vi "GetProbePlanCoordinates.vi"(8 "Use index as X coord":bool=TRUE, 9 "Probe Card Channels":i32=1) -> (0 "file path":string, 2 "OK?":bool, 3 "Array":T1(array[cluster]))   [LabVIEW 2018] (continued)
y=33870.77 \nLabel=Strip\t1026\tX=71822.91\ty=33981.80 \nLabel=Strip\t1027\tX=71468.59\ty=34027.48 \nLabel=Strip\t1028\tX=71811.19\ty=34138.63 \nLabel=Strip\t1029\tX=71456.86\ty=34184.19 \nLabel=Strip\t1030\tX=71799.42\ty=34295.46 \nLabel=Strip\t1031\tX=71445.07\ty=34340.89 \nLabel=Strip\t1032\tX=71787.60\ty=34452.28 \nLabel=Strip\t1033\tX=71433.24\ty=34497.60 \nLabel=Strip\t1034\tX=71775.72\ty=34609.10 \nLabel=Strip\t1035\tX=71421.34\ty=34654.30 \nLabel=Strip\t1036\tX=71763.79\ty=34765.92 \nLabel=Strip\t1037\tX=71409.40\ty=34810.99 \nLabel=Strip\t1038\tX=71751.81\ty=34922.74 \nLabel=Strip\t1039\tX=71397.40\ty=34967.69 \nLabel=Strip\t1040\tX=71739.77\ty=35079.55 \nLabel=Strip\t1041\tX=71385.34\ty=35124.38 \nLabel=Strip\t1042\tX=71727.67\ty=35236.35 \nLabel=Strip\t1043\tX=71373.23\ty=35281.06 \nLabel=Strip\t1044\tX=71715.53\ty=35393.16 \nLabel=Strip\t1045\tX=71361.07\ty=35437.75 \nLabel=Strip\t1046\tX=71703.33\ty=35549.96 \nLabel=Strip\t1047\tX=71348.85\ty=35594.43 \nLabel=Strip\t1048\tX=71691.07\ty=35706.76 \nLabel=Strip\t1049\tX=71336.58\ty=35751.10 \nLabel=Strip\t1050\tX=71678.76\ty=35863.56 \nLabel=Strip\t1051\tX=71324.26\ty=35907.78 \nLabel=Strip\t1052\tX=71666.40\ty=36020.35 \nLabel=Strip\t1053\tX=71311.88\ty=36064.45 \nLabel=Strip\t1054\tX=71653.98\ty=36177.14 \nLabel=Strip\t1055\tX=71299.45\ty=36221.12 \nLabel=Strip\t1056\tX=71641.51\ty=36333.92 \nLabel=Strip\t1057\tX=71286.96\ty=36377.78 \nLabel=Strip\t1058\tX=71628.98\ty=36490.71 \nLabel=Strip\t1059\tX=71274.42\ty=36534.44 \nLabel=Strip\t1060\tX=71616.41\ty=36647.49 \nLabel=Strip\t1061\tX=71261.83\ty=36691.10 \nLabel=Strip\t1062\tX=71603.77\ty=36804.26 \nLabel=Strip\t1063\tX=71249.18\ty=36847.76 \nLabel=Strip\t1064\tX=71591.09\ty=36961.03 \nLabel=Strip\t1065\tX=71236.48\ty=37004.41 \nLabel=Strip\t1066\tX=71578.34\ty=37117.80 \nLabel=Strip\t1067\tX=71223.72\ty=37161.06 \nLabel=Strip\t1068\tX=71565.55\ty=37274.57 \nLabel=Strip\t1069\tX=71210.91\ty=37317.70 \nLabel=Strip\t1070\tX=71552.70\ty=37431.33 \nLabel=Strip\t1071\tX=71198.05\ty=37474.34 \nLabel=Strip\t1072\tX=71539.80\ty=37588.09 \nLabel=Strip\t1073\tX=71185.13\ty=37630.98 \nLabel=Strip\t1074\tX=71526.84\ty=37744.85 \nLabel=Strip\t1075\tX=71172.16\ty=37787.61 \nLabel=Strip\t1076\tX=71513.83\ty=37901.60 \nLabel=Strip\t1077\tX=71159.13\ty=37944.25 \nLabel=Strip\t1078\tX=71500.76\ty=38058.35 \nLabel=Strip\t1079\tX=71146.05\ty=38100.87 \nLabel=Strip\t1080\tX=71487.64\ty=38215.09 \nLabel=Strip\t1081\tX=71132.92\ty=38257.50 \nLabel=Strip\t1082\tX=71474.47\ty=38371.83 \nLabel=Strip\t1083\tX=71119.73\ty=38414.12 \nLabel=Strip\t1084\tX=71461.24\ty=38528.57 \nLabel=Strip\t1085\tX=71106.49\ty=38570.73 \nLabel=Strip\t1086\tX=71447.96\ty=38685.31 \nLabel=Strip\t1087\tX=71093.19\ty=38727.35 \nLabel=Strip\t1088\tX=71434.62\ty=38842.04 \nLabel=Strip\t1089\tX=71079.84\ty=38883.96 \nLabel=Strip\t1090\tX=71421.24\ty=38998.77 \nLabel=Strip\t1091\tX=71066.44\ty=39040.56 \nLabel=Strip\t1092\tX=71407.79\ty=39155.49 \nLabel=Strip\t1093\tX=71052.98\ty=39197.17 \nLabel=Strip\t1094\tX=71394.30\ty=39312.21 \nLabel=Strip\t1095\tX=71039.47\ty=39353.77 \nLabel=Strip\t1096\tX=71380.74\ty=39468.93 \nLabel=Strip\t1097\tX=71025.90\ty=39510.36 \nLabel=Strip\t1098\tX=71367.14\ty=39625.64 \nLabel=Strip\t1099\tX=71012.28\ty=39666.95 \nLabel=Strip\t1100\tX=71353.48\ty=39782.35 \nLabel=Strip\t1101\tX=70998.61\ty=39823.54 \nLabel=Strip\t1102\tX=71339.77\ty=39939.06 \nLabel=Strip\t1103\tX=70984.88\ty=39980.13 \nLabel=Strip\t1104\tX=71326.00\ty=40095.76 \nLabel=Strip\t1105\tX=70971.10\ty=40136.71 \nLabel=Strip\t1106\tX=71312.18\ty=40252.46 \nLabel=Strip\t1107\tX=70957.26\ty=40293.29 \nLabel=Strip\t1108\tX=71298.30\ty=40409.15 \nLabel=Strip\t1109\tX=70943.37\ty=40449.86 \nLabel=Strip\t1110\tX=71284.37\ty=40565.84 \nLabel=Strip\t1111\tX=70929.43\ty=40606.43 \nLabel=Strip\t1112\tX=71270.39\ty=40722.53 \nLabel=Strip\t1113\tX=70915.43\ty=40762.99 \nLabel=Strip\t1114\tX=71256.35\ty=40879.21 \nLabel=Strip\t1115\tX=70901.38\ty=40919.56 \nLabel=Strip\t1116\tX=71242.26\ty=41035.89 \nLabel=Strip\t1117\tX=70887.28\ty=41076.11 \nLabel=Strip\t1118\tX=71228.11\ty=41192.57 \nLabel=Strip\t1119\tX=70873.12\ty=41232.67 \nLabel=Strip\t1120\tX=71213.92\ty=41349.24 \nLabel=Strip\t1121\tX=70858.90\ty=41389.22 \nLabel=Strip\t1122\tX=71199.66\ty=41505.91 \nLabel=Strip\t1123\tX=70844.64\ty=41545.77 \nLabel=Strip\t1124\tX=71185.36\ty=41662.57 \nLabel=Strip\t1125\tX=70830.32\ty=41702.31 \nLabel=Strip\t1126\tX=71170.99\ty=41819.23 \nLabel=Strip\t1127\tX=70815.94\ty=41858.85 \nLabel=Strip\t1128\tX=71156.58\ty=41975.89 \nLabel=Strip\t1129\tX=70801.51\ty=42015.38 \nLabel=Strip\t1130\tX=71142.11\ty=42132.54 \nLabel=Strip\t1131\tX=70787.03\ty=42171.91 \nLabel=Strip\t1132\tX=71127.59\ty=42289.19 \nLabel=Strip\t1133\tX=70772.49\ty=42328.44 \nLabel=Strip\t1134\tX=71113.01\ty=42445.83 \nLabel=Strip\t1135\tX=70757.90\ty=42484.96 \nLabel=Strip\t1136\tX=71098.38\ty=42602.47 \nLabel=Strip\t1137\tX=70743.26\ty=42641.48 \nLabel=Strip\t1138\tX=71083.69\ty=42759.11 \nLabel=Strip\t1139\tX=70728.56\ty=42798.00 \nLabel=Strip\t1140\tX=71068.95\ty=42915.74 \nLabel=Strip\t1141\tX=70713.80\ty=42954.51 \nLabel=Strip\t1142\tX=71054.16\ty=43072.37 \nLabel=Strip\t1143\tX=70699.00\ty=43111.01 \nLabel=Strip\t1144\tX=71039.31\ty=43229.00 \nLabel=Strip\t1145\tX=70684.14\ty=43267.52 \nLabel=Strip\t1146\tX=71024.41\ty=43385.62 \nLabel=Strip\t1147\tX=70669.22\ty=43424.02 \nLabel=Strip\t1148\tX=71009.46\ty=43542.23 \nLabel=Strip\t1149\tX=70654.25\ty=43580.51 \nLabel=Strip\t1150\tX=70994.45\ty=43698.84 \nLabel=Strip\t1151\tX=70639.23\ty=43737.00 \nLabel=Strip\t1152\tX=70979.38\ty=43855.45 \nLabel=Strip\t1153\tX=70624.16\ty=43893.49 \nLabel=Strip\t1154\tX=70964.27\ty=44012.06 \nRegion=Segment\t0T\nLabel=Strip\t1\tX=100771.56\ty=-48853.60 \nLabel=Strip\t2\tX=101128.74\ty=-48799.25 \nLabel=Strip\t3\tX=100788.28\ty=-48687.35 \nLabel=Strip\t4\tX=101145.44\ty=-48632.88 \nLabel=Strip\t5\tX=100804.94\ty=-48521.10 \nLabel=Strip\t6\tX=101162.09\ty=-48466.50 \nLabel=Strip\t7\tX=100821.55\ty=-48354.83 \nLabel=Strip\t8\tX=101178.67\ty=-48300.12 \nLabel=Strip\t9\tX=100838.10\ty=-48188.57 \nLabel=Strip\t10\tX=101195.20\ty=-48133.73 \nLabel=Strip\t11\tX=100854.59\ty=-48022.29 \nLabel=Strip\t12\tX=101211.68\ty=-47967.33 \nLabel=Strip\t13\tX=100871.02\ty=-47856.01 \nLabel=Strip\t14\tX=101228.10\ty=-47800.92 \nLabel=Strip\t15\tX=100887.40\ty=-47689.72 \nLabel=Strip\t16\tX=101244.45\ty=-47634.51 \nLabel=Strip\t17\tX=100903.72\ty=-47523.43 \nLabel=Strip\t18\tX=101260.76\ty=-47468.10 \nLabel=Strip\t19\tX=100919.99\ty=-47357.13 \nLabel=Strip\t20\tX=101277.00\ty=-47301.67 \nLabel=Strip\t21\tX=100936.20\ty=-47190.82 \nLabel=Strip\t22\tX=101293.19\ty=-47135.24 \nLabel=Strip\t23\tX=100952.35\ty=-47024.51 \nLabel=Strip\t24\tX=101309.32\ty=-46968.80 \nLabel=Strip\t25\tX=100968.44\ty=-46858.19 \nLabel=Strip\t26\tX=101325.40\ty=-46802.36 \nLabel=Strip\t27\tX=100984.48\ty=-46691.86 \nLabel=Strip\t28\tX=101341.41\ty=-46635.91 \nLabel=Strip\t29\tX=101000.46\ty=-46525.53 \nLabel=Strip\t30\tX=101357.37\ty=-46469.45 \nLabel=Strip\t31\tX=101016.38\ty=-46359.18 \nLabel=Strip\t32\tX=101373.28\ty=-46302.99 \nLabel=Strip\t33\tX=101032.25\ty=-46192.84 \nLabel=Strip\t34\tX=101389.13\ty=-46136.52 \nLabel=Strip\t35\tX=101048.05\ty=-46026.49 \nLabel=Strip\t36\tX=101404.91\ty=-45970.04 \nLabel=Strip\t37\tX=101063.81\ty=-45860.13 \nLabel=Strip\t38\tX=101420.65\ty=-45803.57 \nLabel=Strip\t39\tX=101079.50\ty=-45693.76 \nLabel=Strip\t40\tX=101436.32\ty=-45637.07 \nLabel=Strip\t41\tX=101095.14\ty=-45527.39 \nLabel=Strip\t42\tX=101451.94\ty=-45470.58 \nLabel=Strip\t43\tX=101110.72\ty=-45361.01 \nLabel=Strip\t44\tX=101467.50\ty=-45304.08 \nLabel=Strip\t45\tX=101126.24\ty=-45194.62 \nLabel=Strip\t46\tX=101483.01\ty=-45137.57 \nLabel=Strip\t47\tX=101141.71\ty=-45028.23 \nLabel=Strip\t48\tX=101498.46\ty=-44971.05 \nLabel=Strip\t49\tX=101157.12\ty=-44861.83 \nLabel=Strip\t50\tX=101513.85\ty=-44804.53 \nLabel=Strip\t51\tX=101172.48\ty=-44695.43 \nLabel=Strip\t52\tX=101529.18\ty=-44638.01 \nLabel=Strip\t53\tX=101187.77\ty=-44529.02 \nLabel=Strip\t54\tX=101544.46\ty=-44471.47 \nLabel=Strip\t55\tX=101203.01\ty=-44362.60 \nLabel=Strip\t56\tX=101559.68\ty=-44304.93 \nLabel=Strip\t57\tX=101218.19\ty=-44196.18 \nLabel=Strip\t58\tX=101574.84\ty=-44138.39 \nLabel=Strip\t59\tX=101233.32\ty=-44029.75 \nLabel=Strip\t60\tX=101589.95\ty=-43971.83 \nLabel=Strip\t61\tX=101248.39\ty=-43863.32 \nLabel=Strip\t62\tX=101604.99\ty=-43805.28 \nLabel=Strip\t63\tX=101263.40\ty=-43696.88 \nLabel=Strip\t64\tX=101619.99\ty=-43638.71 \nLabel=Strip\t65\tX=101278.35\ty=-43530.43 \nLabel=Strip\t66\tX=101634.92\ty=-43472.14 \nLabel=Strip\t67\tX=101293.25\ty=-43363.97 \nLabel=Strip\t68\tX=101649.80\ty=-43305.57 \nLabel=Strip\t69\tX=101308.09\ty=-43197.51 \nLabel=Strip\t70\tX=101664.62\ty=-43138.98 \nLabel=Strip\t71\tX=101322.88\ty=-43031.05 \nLabel=Strip\t72\tX=101679.38\ty=-42972.39 \nLabel=Strip\t73\tX=101337.60\ty=-42864.58 \nLabel=Strip\t74\tX=101694.09\ty=-42805.80 \nLabel=Strip\t75\tX=101352.27\ty=-42698.10 \nLabel=Strip\t76\tX=101708.74\ty=-42639.20 \nLabel=Strip\t77\tX=101366.88\ty=-42531.61 \nLabel=Strip\t78\tX=101723.33\ty=-42472.59 \nLabel=Strip\t79\tX=101381.44\ty=-42365.12 \nLabel=Strip\t80\tX=101737.87\ty=-42305.98 \nLabel=Strip\t81\tX=101395.94\ty=-42198.63 \nLabel=Strip\t82\tX=101752.34\ty=-42139.36 \nLabel=Strip\t83\tX=101410.38\ty=-42032.12 \nLabel=Strip\t84\tX=101766.77\ty=-41972.73 \nLabel=Strip\t85\tX=101424.77\ty=-41865.62 \nLabel=Strip\t86\tX=101781.13\ty=-41806.10 \nLabel=Strip\t87\tX=101439.09\ty=-41699.10 \nLabel=Strip\t88\tX=101795.44\ty=-41639.46 \nLabel=Strip\t89\tX=101453.36\ty=-41532.58 \nLabel=Strip\t90\tX=101809.69\ty=-41472.82 \nLabel=Strip\t91\tX=101467.58\ty=-41366.06 \nLabel=Strip\t92\tX=101823.88\ty=-41306.17 \nLabel=Strip\t93\tX=101481.73\ty=-41199.52 \nLabel=Strip\t94\tX=101838.02\ty=-41139.52 \nLabel=Strip\t95\tX=101495.83\ty=-41032.99 \nLabel=Strip\t96\tX=101852.10\ty=-40972.86 \nLabel=Strip\t97\tX=101509.88\ty=-40866.44 \nLabel=Strip\t98\tX=101866.12\ty=-40806.19 \nLabel=Strip\t99\tX=101523.86\ty=-40699.89 \nLabel=Strip\t100\tX=101880.08\ty=-40639.52 \nLabel=Strip\t101\tX=101537.79\ty=-40533.34 \nLabel=Strip\t102\tX=101893.99\ty=-40472.84 \nLabel=Strip\t103\tX=101551.66\ty=-40366.78 \nLabel=Strip\t104\tX=101907.84\ty=-40306.16 \nLabel=Strip\t105\tX=101565.48\ty=-40200.21 \nLabel=Strip\t106\tX=101921.64\ty=-40139.47 \nLabel=Strip\t107\tX=101579.23\ty=-40033.64 \nLabel=Strip\t108\tX=101935.37\ty=-39972.77 \nLabel=Strip\t109\tX=101592.93\ty=-39867.06 \nLabel=Strip\t110\tX=101949.05\ty=-39806.07 \nLabel=Strip\t111\tX=101606.58\ty=-39700.48 \nLabel=Strip\t112\tX=101962.67\ty=-39639.36 \nLabel=Strip\t113\tX=101620.16\ty=-39533.89 \nLabel=Strip\t114\tX=101976.24\ty=-39472.65 \nLabel=Strip\t115\tX=101633.69\ty=-39367.29 \nLabel=Strip\t116\tX=101989.75\ty=-39305.93 \nLabel=Strip\t117\tX=101647.16\ty=-39200.69 \nLabel=Strip\t118\tX=102003.20\ty=-39139.21 \nLabel=Strip\t119\tX=101660.58\ty=-39034.08 \nLabel=Strip\t120\tX=102016.59\ty=-38972.48 \nLabel=Strip\t121\tX=101673.94\ty=-38867.47 \nLabel=Strip\t122\tX=102029.93\ty=-38805.74 \nLabel=Strip\t123\tX=101687.24\ty=-38700.85 \nLabel=Strip\t124\tX=102043.21\ty=-38639.00 \nLabel=Strip\t125\tX=101700.48\ty=-38534.23 \nLabel=Strip\t126\tX=102056.43\ty=-38472.26 \nLabel=Strip\t127\tX=101713.67\ty=-38367.60 \nLabel=Strip\t128\tX=102069.60\ty=-38305.51 \nLabel=Strip\t129\tX=101726.80\ty=-38200.97 \nLabel=Strip\t130\tX=102082.71\ty=-38138.75 \nLabel=Strip\t131\tX=101739.87\ty=-38034.33 \nLabel=Strip\t132\tX=102095.76\ty=-37971.99 \nLabel=Strip\t133\tX=101752.89\ty=-37867.68 \nLabel=Strip\t134\tX=102108.75\ty=-37805.22 \nLabel=Strip\t135\tX=101765.85\ty=-37701.03 \nLabel=Strip\t136\tX=102121.69\ty=-37638.44 \nLabel=Strip\t137\tX=101778.75\ty=-37534.37 \nLabel=Strip\t138\tX=102134.57\ty=-37471.66 \nLabel=Strip\t139\tX=101791.59\ty=-37367.71 \nLabel=Strip\t140\tX=102147.39\ty=-37304.88 \nLabel=Strip\t141\tX=101804.38\ty=-37201.04 \nLabel=Strip\t142\tX=102160.16\ty=-37138.09 \nLabel=Strip\t143\tX=101817.11\ty=-37034.37 \nLabel=Strip\t144\tX=102172.87\ty=-36971.29 \nLabel=Strip\t145\tX=101829.78\ty=-36867.69 \nLabel=Strip\t146\tX=102185.52\ty=-36804.49 \nLabel=Strip\t147\tX=101842.40\ty=-36701.01 \nLabel=Strip\t148\tX=102198.11\ty=-36637.69 \nLabel=Strip\t149\tX=101854.96\ty=-36534.32 \nLabel=Strip\t150\tX=102210.65\ty=-36470.88 \nLabel=Strip\t151\tX=101867.46\ty=-36367.62 \nLabel=Strip\t152\tX=102223.13\ty=-36304.06 \nLabel=Strip\t153\tX=101879.91\ty=-36200.92 \nLabel=Strip\t154\tX=102235.55\ty=-36137.24 \nLabel=Strip\t155\tX=101892.29\ty=-36034.22 \nLabel=Strip\t156\tX=102247.92\ty=-35970.41 \nLabel=Strip\t157\tX=101904.62\ty=-35867.51 \nLabel=Strip\t158\tX=102260.23\ty=-35803.58 \nLabel=Strip\t159\tX=101916.90\ty=-35700.79 \nLabel=Strip\t160\tX=102272.48\ty=-35636.74 \nLabel=Strip\t161\tX=101929.11\ty=-35534.07 \nLabel=Strip\t162\tX=102284.67\ty=-35469.89 \nLabel=Strip\t163\tX=101941.27\ty=-35367.35 \nLabel=Strip\t164\tX=102296.81\ty=-35303.05 \nLabel=Strip\t165\tX=101953.38\ty=-35200.62 \nLabel=Strip\t166\tX=102308.89\ty=-35136.19 \nLabel=Strip\t167\tX=101965.42\ty=-35033.88 \nLabel=Strip\t168\tX=102320.91\ty=-34969.33 \nLabel=Strip\t169\tX=101977.41\ty=-34867.14 \nLabel=Strip\t170\tX=102332.88\ty=-34802.47 \nLabel=Strip\t171\tX=101989.34\ty=-34700.39 \nLabel=Strip\t172\tX=102344.79\ty=-34635.60 \nLabel=Strip\t173\tX=102001.21\ty=-34533.64 \nLabel=Strip\t174\tX=102356.64\ty=-34468.74 \nLabel=Strip\t175\tX=102013.03\ty=-34366.88 \nLabel=Strip\t176\tX=102368.43\ty=-34301.85 \nLabel=Strip\t177\tX=102024.79\ty=-34200.12 \nLabel=Strip\t178\tX=102380.17\ty=-34134.96 \nLabel=Strip\t179\tX=102036.49\ty=-34033.36 \nLabel=Strip\t180\tX=102391.85\ty=-33968.07 \nLabel=Strip\t181\tX=102048.14\ty=-33866.58 \nLabel=Strip\t182\tX=102403.48\ty=-33801.18 \nLabel=Strip\t183\tX=102059.72\ty=-33699.81 \nLabel=Strip\t184\tX=102415.04\ty=-33634.28 \nLabel=Strip\t185\tX=102071.26\ty=-33533.03 \nLabel=Strip\t186\tX=102426.55\ty=-33467.38 \nLabel=Strip\t187\tX=102082.73\ty=-33366.24 \nLabel=Strip\t188\tX=102438.00\ty=-33300.47 \nLabel=Strip\t189\tX=102094.15\ty=-33199.45 \nLabel=Strip\t190\tX=102449.39\ty=-33133.55 \nLabel=Strip\t191\tX=102105.50\ty=-33032.65 \nLabel=Strip\t192\tX=102460.73\ty=-32966.63 \nLabel=Strip\t193\tX=102116.81\ty=-32865.85 \nLabel=Strip\t194\tX=102472.01\ty=-32799.71 \nLabel=Strip\t195\tX=102128.05\ty=-32699.04 \nLabel=Strip\t196\tX=102483.23\ty=-32632.78 \nLabel=Strip\t197\tX=102139.24\ty=-32532.23 \nLabel=Strip\t198\tX=102494.40\ty=-32465.85 \nLabel=Strip\t199\tX=102150.37\ty=-32365.42 \nLabel=Strip\t200\tX=102505.51\ty=-32298.91 \nLabel=Strip\t201\tX=102161.45\ty=-32198.59 \nLabel=Strip\t202\tX=102516.56\ty=-32131.96 \nLabel=Strip\t203\tX=102172.46\ty=-32031.77 \nLabel=Strip\t204\tX=102527.55\ty=-31965.02 \nLabel=Strip\t205\tX=102183.42\ty=-31864.94 \nLabel=Strip\t206\tX=102538.49\ty=-31798.06 \nLabel=Strip\t207\tX=102194.32\ty=-31698.10 \nLabel=Strip\t208\tX=102549.37\ty=-31631.10 \nLabel=Strip\t209\tX=102205.17\ty=-31531.26 \nLabel=Strip\t210\tX=102560.19\ty=-31464.14 \nLabel=Strip\t211\tX=102215.96\ty=-31364.42 \nLabel=Strip\t212\tX=102570.96\ty=-31297.17 \nLabel=Strip\t213\tX=102226.69\ty=-31197.57 \nLabel=Strip\t214\tX=102581.66\ty=-31130.20 \nLabel=Strip\t215\tX=102237.36\ty=-31030.71 \nLabel=Strip\t216\tX=102592.31\ty=-30963.23 \nLabel=Strip\t217\tX=102247.98\ty=-30863.85 \nLabel=Strip\t218\tX=102602.91\ty=-30796.24 \nLabel=Strip\t219\tX=102258.54\ty=-30696.99 \nLabel=Strip\t220\tX=102613.44\ty=-30629.26 \nLabel=Strip\t221\tX=102269.04\ty=-30530.12 \nLabel=Strip\t222\tX=102623.92\ty=-30462.27 \nLabel=Strip\t223\tX=102279.48\ty=-30363.25 \nLabel=Strip\t224\tX=102634.34\ty=-30295.27 \nLabel=Strip\t225\tX=102289.87\ty=-30196.37 \nLabel=Strip\t226\tX=102644.71\ty=-30128.27 \nLabel=Strip\t227\tX=102300.20\ty=-30029.49 \nLabel=Strip\t228\tX=102655.02\ty=-29961.27 \nLabel=Strip\t229\tX=102310.48\ty=-29862.60 \nLabel=Strip\t230\tX=102665.27\ty=-29794.26 \nLabel=Strip\t231\tX=102320.69\ty=-29695.71 \nLabel=Strip\t232\tX=102675.46\ty=-29627.24 \nLabel=Strip\t233\tX=102330.85\ty=-29528.81 \nLabel=Strip\t234\tX=102685.59\ty=-29460.23 \nLabel=Strip\t235\tX=102340.95\ty=-29361.91 \nLabel=Strip\t236\tX=102695.67\ty=-29293.20 \nLabel=Strip\t237\tX=102351.00\ty=-29195.01 \nLabel=Strip\t238\tX=102705.69\ty=-29126.18 \nLabel=Strip\t239\tX=102360.99\ty=-29028.10 \nLabel=Strip\t240\tX=102715.66\ty=-28959.14 \nLabel=Strip\t241\tX=102370.91\ty=-28861.19 \nLabel=Strip\t242\tX=102725.56\ty=-28792.11 \nLabel=Strip\t243\tX=102380.79\ty=-28694.27 \nLabel=Strip\t244\tX=102735.41\ty=-28625.07 \nLabel=Strip\t245\tX=102390.60\ty=-28527.34 \nLabel=Strip\t246\tX=102745.20\ty=-28458.02 \nLabel=Strip\t247\tX=102400.36\ty=-28360.42 \nLabel=Strip\t248\tX=102754.94\ty=-28290.97 \nLabel=Strip\t249\tX=102410.06\ty=-28193.49 \nLabel=Strip\t250\tX=102764.62\ty=-28123.92 \nLabel=Strip\t251\tX=102419.71\ty=-28026.55 \nLabel=Strip\t252\tX=102774.24\ty=-27956.86 \nLabel=Strip\t253\tX=102429.29\ty=-27859.61 \nLabel=Strip\t254\tX=102783.80\ty=-27789.80 \nLabel=Strip\t255\tX=102438.82\ty=-27692.67 \nLabel=Strip\t256\tX=102793.31\ty=-27622.73 \nLabel=Strip\t257\tX=102448.30\ty=-27525.72 \nLabel=Strip\t258\tX=102802.75\ty=-27455.66 \nLabel=Strip\t259\tX=102457.71\ty=-27358.76 \nLabel=Strip\t260\tX=102812.15\ty=-27288.59 \nLabel=Strip\t261\tX=102467.07\ty=-27191.81 \nLabel=Strip\t262\tX=102821.48\ty=-27121.51 \nLabel=Strip\t263\tX=102476.37\ty=-27024.85 \nLabel=Strip\t264\tX=102830.76\ty=-26954.42 \nLabel=Strip\t265\tX=102485.61\ty=-26857.88 \nLabel=Strip\t266\tX=102839.98\ty=-26787.34 \nLabel=Strip\t267\tX=102494.80\ty=-26690.91 \nLabel=Strip\t268\tX=102849.14\ty=-26620.24 \nLabel=Strip\t269\tX=102503.93\ty=-26523.94 \nLabel=Strip\t270\tX=102858.24\ty=-26453.15 \nLabel=Strip\t271\tX=102513.00\ty=-26356.96 \nLabel=Strip\t272\tX=102867.29\ty=-26286.05 \nLabel=Strip\t273\tX=102522.02\ty=-26189.98 \nLabel=Strip\t274\tX=102876.28\ty=-26118.94 \nLabel=Strip\t275\tX=102530.97\ty=-26022.99 \nLabel=Strip\t276\tX=102885.21\ty=-25951.83 \nLabel=Strip\t277\tX=102539.87\ty=-25856.00 \nLabel=Strip\t278\tX=102894.09\ty=-25784.72 \nLabel=Strip\t279\tX=102548.73\ty=-25688.73 \nLabel=Strip\t280\tX=102902.91\ty=-25617.61 \nLabel=Strip\t281\tX=102557.50\ty=-25522.01 \nLabel=Strip\t282\tX=102911.67\ty=-25450.48 \nLabel=Strip\t283\tX=102566.23\ty=-25355.00 \nLabel=Strip\t284\tX=102920.37\ty=-25283.36 \nLabel=Strip\t285\tX=102574.90\ty=-25188.00 \nLabel=Strip\t286\tX=102929.02\ty=-25116.23 \nLabel=Strip\t287\tX=102583.52\ty=-25020.99 \nLabel=Strip\t288\tX=102937.61\ty=-24949.10 \nLabel=Strip\t289\tX=102592.07\ty=-24853.97 \nLabel=Strip\t290\tX=102946.14\ty=-24781.96 \nLabel=Strip\t291\tX=102600.57\ty=-24686.95 \nLabel=Strip\t292\tX=102954.62\ty=-24614.82 \nLabel=Strip\t293\tX=102609.02\ty=-24519.93 \nLabel=Strip\t294\tX=102963.03\ty=-24447.68 \nLabel=Strip\t295\tX=102617.40\ty=-24352.90 \nLabel=Strip\t296\tX=102971.39\ty=-24280.53 \nLabel=Strip\t297\tX=102625.73\ty=-24185.87 \nLabel=Strip\t298\tX=102979.70\ty=-24113.37 \nLabel=Strip\t299\tX=102634.00\ty=-24018.84 \nLabel=Strip\t300\tX=102987.94\ty=-23946.22 \nLabel=Strip\t301\tX=102642.21\ty=-23851.80 \nLabel=Strip\t302\tX=102996.13\ty=-23779.06 \nLabel=Strip\t303\tX=102650.37\ty=-23684.76 \nLabel=Strip\t304\tX=103004.26\ty=-23611.89 \nLabel=Strip\t305\tX=102658.47\ty=-23517.71 \nLabel=Strip\t306\tX=103012.33\ty=-23444.73 \nLabel=Strip\t307\tX=102666.51\ty=-23350.66 \nLabel=Strip\t308\tX=103020.35\ty=-23277.56 \nLabel=Strip\t309\tX=102674.49\ty=-23183.61 \nLabel=Strip\t310\tX=103028.31\ty=-23110.38 \nLabel=Strip\t311\tX=102682.42\ty=-23016.55 \nLabel=Strip\t312\tX=103036.21\ty=-22943.20 \nLabel=Strip\t313\tX=102690.29\ty=-22849.49 \nLabel=Strip\t314\tX=103044.06\ty=-22776.02 \nLabel=Strip\t315\tX=102698.10\ty=-22682.43 \nLabel=Strip\t316\tX=103051.84\ty=-22608.83 \nLabel=Strip\t317\tX=102705.85\ty=-22515.36 \nLabel=Strip\t318\tX=103059.57\ty=-22441.64 \nLabel=Strip\t319\tX=102713.55\ty=-22348.29 \nLabel=Strip\t320\tX=103067.24\ty=-22274.45 \nLabel=Strip\t321\tX=102721.19\ty=-22181.21 \nLabel=Strip\t322\tX=103074.86\ty=-22107.25 \nLabel=Strip\t323\tX=102728.78\ty=-22014.13 \nLabel=Strip\t324\tX=103082.42\ty=-21940.05 \nLabel=Strip\t325\tX=102736.30\ty=-21847.05 \nLabel=Strip\t326\tX=103089.92\ty=-21772.84 \nLabel=Strip\t327\tX=102743.77\ty=-21679.96 \nLabel=Strip\t328\tX=103097.36\ty=-21605.63 \nLabel=Strip\t329\tX=102751.18\ty=-21512.87 \nLabel=Strip\t330\tX=103104.75\ty=-21438.42 \nLabel=Strip\t331\tX=102758.53\ty=-21345.78 \nLabel=Strip\t332\tX=103112.08\ty=-21271.21 \nLabel=Strip\t333\tX=102765.83\ty=-21178.68 \nLabel=Strip\t334\tX=103119.35\ty=-21103.99 \nLabel=Strip\t335\tX=102773.07\ty=-21011.58 \nLabel=Strip\t336\tX=103126.56\ty=-20936.77 \nLabel=Strip\t337\tX=102780.25\ty=-20844.48 \nLabel=Strip\t338\tX=103133.72\ty=-20769.54 \nLabel=Strip\t339\tX=102787.38\ty=-20677.37 \nLabel=Strip\t340\tX=103140.82\ty=-20602.31 \nLabel=Strip\t341\tX=102794.45\ty=-20510.26 \nLabel=Strip\t342\tX=103147.86\ty=-20435.08 \nLabel=Strip\t343\tX=102801.45\ty=-20343.14 \nLabel=Strip\t344\tX=103154.84\ty=-20267.84 \nLabel=Strip\t345\tX=102808.41\ty=-20176.03 \nLabel=Strip\t346\tX=103161.77\ty=-20100.60 \nLabel=Strip\t347\tX=102815.30\ty=-20008.90 \nLabel=Strip\t348\tX=103168.64\ty=-19933.36 \nLabel=Strip\t349\tX=102822.14\ty=-19841.78 \nLabel=Strip\t350\tX=103175.45\ty=-19766.11 \nLabel=Strip\t351\tX=102828.92\ty=-19674.65 \nLabel=Strip\t352\tX=103182.20\ty=-19598.86 \nLabel=Strip\t353\tX=102835.65\ty=-19507.52 \nLabel=Strip\t354\tX=103188.90\ty=-19431.61 \nLabel=Strip\t355\tX=102842.31\ty=-19340.38 \nLabel=Strip\t356\tX=103195.54\ty=-19264.35 \nLabel=Strip\t357\tX=102848.92\ty=-19173.25 \nLabel=Strip\t358\tX=103202.13\ty=-19097.09 \nLabel=Strip\t359\tX=102855.47\ty=-19006.10 \nLabel=Strip\t360\tX=103208.65\ty=-18929.83 \nLabel=Strip\t361\tX=102861.97\ty=-18838.96 \nLabel=Strip\t362\tX=103215.12\ty=-18762.56 \nLabel=Strip\t363\tX=102868.40\ty=-18671.81 \nLabel=Strip\t364\tX=103221.53\ty=-18595.29 \nLabel=Strip\t365\tX=102874.78\ty=-18504.66 \nLabel=Strip\t366\tX=103227.88\ty=-18428.02 \nLabel=Strip\t367\tX=102881.11\ty=-18337.51 \nLabel=Strip\t368\tX=103234.18\ty=-18260.74 \nLabel=Strip\t369\tX=102887.37\ty=-18170.35 \nLabel=Strip\t370\tX=103240.42\ty=-18093.41 \nLabel=Strip\t371\tX=102893.58\ty=-18003.19 \nLabel=Strip\t372\tX=103246.60\ty=-17926.18 \nLabel=Strip\t373\tX=102899.73\ty=-17836.02 \nLabel=Strip\t374\tX=103252.72\ty=-17758.89 \nLabel=Strip\t375\tX=102905.82\ty=-17668.86 \nLabel=Strip\t376\tX=103258.79\ty=-17591.60 \nLabel=Strip\t377\tX=102911.86\ty=-17501.69 \nLabel=Strip\t378\tX=103264.80\ty=-17424.31 \nLabel=Strip\t379\tX=102917.84\ty=-17334.51 \nLabel=Strip\t380\tX=103270.75\ty=-17257.02 \nLabel=Strip\t381\tX=102923.76\ty=-17167.34 \nLabel=Strip\t382\tX=103276.64\ty=-17089.72 \nLabel=Strip\t383\tX=102929.62\ty=-17000.16 \nLabel=Strip\t384\tX=103282.48\ty=-16922.42 \nLabel=Strip\t385\tX=102935.43\ty=-16832.97 \nLabel=Strip\t386\tX=103288.26\ty=-16755.11 \nLabel=Strip\t387\tX=102941.18\ty=-16665.79 \nLabel=Strip\t388\tX=103293.98\ty=-16587.81 \nLabel=Strip\t389\tX=102946.87\ty=-16498.60 \nLabel=Strip\t390\tX=103299.65\ty=-16420.50 \nLabel=Strip\t391\tX=102952.50\ty=-16331.41 \nLabel=Strip\t392\tX=103305.26\ty=-16253.18 \nLabel=Strip\t393\tX=102958.08\ty=-16164.21 \nLabel=Strip\t394\tX=103310.81\ty=-16085.87 \nLabel=Strip\t395\tX=102963.60\ty=-15997.02 \nLabel=Strip\t396\tX=103316.30\ty=-15918.55 \nLabel=Strip\t397\tX=102969.06\ty=-15829.82 \nLabel=Strip\t398\tX=103321.73\ty=-15751.23 \nLabel=Strip\t399\tX=102974.46\ty=-15662.61 \nLabel=Strip\t400\tX=103327.11\ty=-15583.90 \nLabel=Strip\t401\tX=102979.81\ty=-15495.41 \nLabel=Strip\t402\tX=103332.43\ty=-15416.57 \nLabel=Strip\t403\tX=102985.10\ty=-15328.20 \nLabel=Strip\t404\tX=103337.69\ty=-15249.24 \nLabel=Strip\t405\tX=102990.33\ty=-15160.99 \nLabel=Strip\t406\tX=103342.90\ty=-15081.91 \nLabel=Strip\t407\tX=102995.51\ty=-14993.77 \nLabel=Strip\t408\tX=103348.05\ty=-14914.57 \nLabel=Strip\t409\tX=103000.63\ty=-14826.55 \nLabel=Strip\t410\tX=103353.14\ty=-14747.23 \nLabel=Strip\t411\tX=103005.69\ty=-14659.33 \nLabel=Strip\t412\tX=103358.17\ty=-14579.89 \nLabel=Strip\t413\tX=103010.69\ty=-14492.11 \nLabel=Strip\t414\tX=103363.15\ty=-14412.55 \nLabel=Strip\t415\tX=103015.64\ty=-14324.88 \nLabel=Strip\t416\tX=103368.07\ty=-14245.20 \nLabel=Strip\t417\tX=103020.53\ty=-14157.66 \nLabel=Strip\t418\tX=103372.93\ty=-14077.85 \nLabel=Strip\t419\tX=103025.36\ty=-13990.42 \nLabel=Strip\t420\tX=103377.73\ty=-13910.50 \nLabel=Strip\t421\tX=103030.13\ty=-13823.19 \nLabel=Strip\t422\tX=103382.48\ty=-13743.14 \nLabel=Strip\t423\tX=103034.85\ty=-13655.95 \nLabel=Strip\t424\tX=103387.17\ty=-13575.78 \nLabel=Strip\t425\tX=103039.51\ty=-13488.72 \nLabel=Strip\t426\tX=103391.80\ty=-13408.42 \nLabel=Strip\t427\tX=103044.11\ty=-13321.47 \nLabel=Strip\t428\tX=103396.37\ty=-13241.06 \nLabel=Strip\t429\tX=103048.65\ty=-13154.23 \nLabel=Strip\t430\tX=103400.89\ty=-13073.69 \nLabel=Strip\t431\tX=103053.14\ty=-12986.98 \nLabel=Strip\t432\tX=103405.35\ty=-12906.33 \nLabel=Strip\t433\tX=103057.57\ty=-12819.73 \nLabel=Strip\t434\tX=103409.75\ty=-12738.96 \nLabel=Strip\t435\tX=103061.94\ty=-12652.48 \nLabel=Strip\t436\tX=103414.10\ty=-12571.58 \nLabel=Strip\t437\tX=103066.26\ty=-12485.23 \nLabel=Strip\t438\tX=103418.38\ty=-12404.21 \nLabel=Strip\t439\tX=103070.51\ty=-12317.97 \nLabel=Strip\t440\tX=103422.61\ty=-12236.83 \nLabel=Strip\t441\tX=103074.71\ty=-12150.71 \nLabel=Strip\t442\tX=103426.78\ty=-12069.45 \nLabel=Strip\t443\tX=103078.86\ty=-11983.45 \nLabel=Strip\t444\tX=103430.90\ty=-11902.06 \nLabel=Strip\t445\tX=103082.94\ty=-11816.18 \nLabel=Strip\t446\tX=103434.96\ty=-11734.68 \nLabel=Strip\t447\tX=103086.97\ty=-11648.92 \nLabel=Strip\t448\tX=103438.96\ty=-11567.29 \nLabel=Strip\t449\tX=103090.94\ty=-11481.65 \nLabel=Strip\t450\tX=103442.90\ty=-11399.90 \nLabel=Strip\t451\tX=103094.85\ty=-11314.38 \nLabel=Strip\t452\tX=103446.78\ty=-11232.50 \nLabel=Strip\t453\tX=103098.71\ty=-11147.10 \nLabel=Strip\t454\tX=103450.61\ty=-11065.11 \nLabel=Strip\t455\tX=103102.51\ty=-10979.82 \nLabel=Strip\t456\tX=103454.49\ty=-10870.83 \nLabel=Strip\t457\tX=103106.33\ty=-10791.27 \nLabel=Strip\t458\tX=103458.15\ty=-10714.16 \nLabel=Strip\t459\tX=103109.97\ty=-10634.60 \nLabel=Strip\t460\tX=103461.77\ty=-10557.49 \nLabel=Strip\t461\tX=103113.56\ty=-10477.93 \nLabel=Strip\t462\tX=103465.33\ty=-10400.82 \nLabel=Strip\t463\tX=103117.09\ty=-10321.26 \nLabel=Strip\t464\tX=103468.83\ty=-10244.14 \nLabel=Strip\t465\tX=103120.57\ty=-10164.58 \nLabel=Strip\t466\tX=103472.29\ty=-10087.47 \nLabel=Strip\t467\tX=103124.09\ty=-9976.12 \nLabel=Strip\t468\tX=103475.79\ty=-9893.28 \nLabel=Strip\t469\tX=103127.48\ty=-9808.83 \nLabel=Strip\t470\tX=103479.16\ty=-9725.86 \nLabel=Strip\t471\tX=103130.82\ty=-9641.53 \nLabel=Strip\t472\tX=103482.47\ty=-9558.45 \nLabel=Strip\t473\tX=103134.11\ty=-9474.23 \nLabel=Strip\t474\tX=103485.72\ty=-9391.03 \nLabel=Strip\t475\tX=103137.33\ty=-9306.94 \nLabel=Strip\t476\tX=103488.92\ty=-9223.61 \nLabel=Strip\t477\tX=103140.50\ty=-9139.64 \nLabel=Strip\t478\tX=103492.06\ty=-9056.19 \nLabel=Strip\t479\tX=103143.61\ty=-8972.33 \nLabel=Strip\t480\tX=103495.14\ty=-8888.76 \nLabel=Strip\t481\tX=103146.66\ty=-8805.03 \nLabel=Strip\t482\tX=103498.16\ty=-8721.34 \nLabel=Strip\t483\tX=103149.65\ty=-8637.72 \nLabel=Strip\t484\tX=103501.13\ty=-8553.91 \nLabel=Strip\t485\tX=103152.59\ty=-8470.41 \nLabel=Strip\t486\tX=103504.04\ty=-8386.48 \nLabel=Strip\t487\tX=103155.47\ty=-8303.10 \nLabel=Strip\t488\tX=103506.89\ty=-8219.05 \nLabel=Strip\t489\tX=103158.29\ty=-8135.79 \nLabel=Strip\t490\tX=103509.68\ty=-8051.61 \nLabel=Strip\t491\tX=103161.06\ty=-7968.47 \nLabel=Strip\t492\tX=103512.42\ty=-7884.17 \nLabel=Strip\t493\tX=103163.76\ty=-7801.15 \nLabel=Strip\t494\tX=103515.09\ty=-7716.74 \nLabel=Strip\t495\tX=103166.41\ty=-7633.83 \nLabel=Strip\t496\tX=103517.71\ty=-7549.30 \nLabel=Strip\t497\tX=103169.00\ty=-7466.51 \nLabel=Strip\t498\tX=103520.28\ty=-7381.85 \nLabel=Strip\t499\tX=103171.54\ty=-7299.19 \nLabel=Strip\t500\tX=103522.78\ty=-7214.41 \nLabel=Strip\t501\tX=103174.02\ty=-7131.86 \nLabel=Strip\t502\tX=103525.23\ty=-7046.96 \nLabel=Strip\t503\tX=103176.44\ty=-6964.54 \nLabel=Strip\t504\tX=103527.62\ty=-6879.51 \nLabel=Strip\t505\tX=103178.80\ty=-6797.21 \nLabel=Strip\t506\tX=103529.96\ty=-6712.07 \nLabel=Strip\t507\tX=103181.10\ty=-6629.88 \nLabel=Strip\t508\tX=103532.23\ty=-6544.61 \nLabel=Strip\t509\tX=103183.35\ty=-6462.55 \nLabel=Strip\t510\tX=103534.45\ty=-6377.16 \nLabel=Strip\t511\tX=103185.54\ty=-6295.21 \nLabel=Strip\t512\tX=103536.61\ty=-6209.71 \nLabel=Strip\t513\tX=103187.68\ty=-6127.88 \nLabel=Strip\t514\tX=103538.71\ty=-6042.25 \nLabel=Strip\t515\tX=103189.75\ty=-5960.54 \nLabel=Strip\t516\tX=103540.76\ty=-5874.79 \nLabel=Strip\t517\tX=103191.77\ty=-5793.20 \nLabel=Strip\t518\tX=103542.75\ty=-5707.33 \nLabel=Strip\t519\tX=103193.73\ty=-5625.86 \nLabel=Strip\t520\tX=103544.68\ty=-5539.87 \nLabel=Strip\t521\tX=103195.63\ty=-5458.52 \nLabel=Strip\t522\tX=103546.55\ty=-5372.40 \nLabel=Strip\t523\tX=103197.48\ty=-5291.17 \nLabel=Strip\t524\tX=103548.37\ty=-5204.94 \nLabel=Strip\t525\tX=103199.27\ty=-5123.82 \nLabel=Strip\t526\tX=103550.13\ty=-5037.47 \nLabel=Strip\t527\tX=103201.00\ty=-4956.48 \nLabel=Strip\t528\tX=103551.83\ty=-4870.00 \nLabel=Strip\t529\tX=103202.67\ty=-4789.13 \nLabel=Strip\t530\tX=103553.47\ty=-4702.53 \nLabel=Strip\t531\tX=103204.29\ty=-4621.78 \nLabel=Strip\t532\tX=103555.06\ty=-4535.06 \nLabel=Strip\t533\tX=103205.85\ty=-4454.42 \nLabel=Strip\t534\tX=103556.59\ty=-4367.59 \nLabel=Strip\t535\tX=103207.35\ty=-4287.07 \nLabel=Strip\t536\tX=103558.06\ty=-4200.11 \nLabel=Strip\t537\tX=103208.79\ty=-4119.71 \nLabel=Strip\t538\tX=103559.47\ty=-4032.63 \nLabel=Strip\t539\tX=103210.18\ty=-3952.36 \nLabel=Strip\t540\tX=103560.83\ty=-3865.16 \nLabel=Strip\t541\tX=103211.50\ty=-3785.00 \nLabel=Strip\t542\tX=103562.13\ty=-3697.68 \nLabel=Strip\t543\tX=103212.77\ty=-3617.64 \nLabel=Strip\t544\tX=103563.37\ty=-3530.19 \nLabel=Strip\t545\tX=103213.99\ty=-3450.28 \nLabel=Strip\t546\tX=103564.55\ty=-3362.71 \nLabel=Strip\t547\tX=103215.14\ty=-3282.91 \nLabel=Strip\t548\tX=103565.68\ty=-3195.23 \nLabel=Strip\t549\tX=103216.24\ty=-3115.55 \nLabel=Strip\t550\tX=103566.75\ty=-3027.74 \nLabel=Strip\t551\tX=103217.28\ty=-2948.18 \nLabel=Strip\t552\tX=103567.76\ty=-2860.20 \nLabel=Strip\t553\tX=103218.27\ty=-2780.81 \nLabel=Strip\t554\tX=103568.71\ty=-2692.77 \nLabel=Strip\t555\tX=103219.20\ty=-2613.45 \nLabel=Strip\t556\tX=103569.61\ty=-2525.28 \nLabel=Strip\t557\tX=103220.06\ty=-2446.07 \nLabel=Strip\t558\tX=103570.45\ty=-2357.79 \nLabel=Strip\t559\tX=103220.87\ty=-2278.70 \nLabel=Strip\t560\tX=103571.23\ty=-2190.29 \nLabel=Strip\t561\tX=103221.63\ty=-2111.33 \nLabel=Strip\t562\tX=103571.95\ty=-2022.80 \nLabel=Strip\t563\tX=103222.33\ty=-1943.96 \nLabel=Strip\t564\tX=103572.62\ty=-1855.31 \nLabel=Strip\t565\tX=103222.96\ty=-1776.58 \nLabel=Strip\t566\tX=103573.23\ty=-1687.81 \nLabel=Strip\t567\tX=103223.55\ty=-1609.21 \nLabel=Strip\t568\tX=103573.78\ty=-1520.31 \nLabel=Strip\t569\tX=103224.07\ty=-1441.83 \nLabel=Strip\t570\tX=103574.27\ty=-1352.81 \nLabel=Strip\t571\tX=103224.54\ty=-1274.45 \nLabel=Strip\t572\tX=103574.71\ty=-1185.32 \nLabel=Strip\t573\tX=103224.94\ty=-1107.07 \nLabel=Strip\t574\tX=103575.08\ty=-1017.81 \nLabel=Strip\t575\tX=103225.30\ty=-939.69 \nLabel=Strip\t576\tX=103575.40\ty=-850.31 \nLabel=Strip\t577\tX=103225.59\ty=-772.31 \nLabel=Strip\t578\tX=103575.67\ty=-682.81 \nLabel=Strip\t579\tX=103225.83\ty=-604.92 \nLabel=Strip\t580\tX=103575.87\ty=-515.31 \nLabel=Strip\t581\tX=103226.01\ty=-437.54 \nLabel=Strip\t582\tX=103576.02\ty=-347.80 \nLabel=Strip\t583\tX=103226.13\ty=-270.15 \nLabel=Strip\t584\tX=103576.11\ty=-180.29 \nLabel=Strip\t585\tX=103226.19\ty=-102.76 \nLabel=Strip\t586\tX=103576.15\ty=-12.79 \nLabel=Strip\t587\tX=103226.20\ty=64.62 \nLabel=Strip\t588\tX=103576.12\ty=154.72 \nLabel=Strip\t589\tX=103226.15\ty=232.01 \nLabel=Strip\t590\tX=103576.04\ty=322.23 \nLabel=Strip\t591\tX=103226.04\ty=399.40 \nLabel=Strip\t592\tX=103575.90\ty=489.74 \nLabel=Strip\t593\tX=103225.87\ty=566.79 \nLabel=Strip\t594\tX=103575.70\ty=657.25 \nLabel=Strip\t595\tX=103225.65\ty=734.18 \nLabel=Strip\t596\tX=103575.45\ty=824.77 \nLabel=Strip\t597\tX=103225.37\ty=901.58 \nLabel=Strip\t598\tX=103575.14\ty=992.28 \nLabel=Strip\t599\tX=103225.03\ty=1068.97 \nLabel=Strip\t600\tX=103574.77\ty=1159.79 \nLabel=Strip\t601\tX=103224.64\ty=1236.37 \nLabel=Strip\t602\tX=103574.34\ty=1327.31 \nLabel=Strip\t603\tX=103224.18\ty=1403.76 \nLabel=Strip\t604\tX=103573.86\ty=1494.83 \nLabel=Strip\t605\tX=103223.67\ty=1571.16 \nLabel=Strip\t606\tX=103573.31\ty=1662.34 \nLabel=Strip\t607\tX=103223.10\ty=1738.55 \nLabel=Strip\t608\tX=103572.71\ty=1829.86 \nLabel=Strip\t609\tX=103222.48\ty=1905.95 \nLabel=Strip\t610\tX=103572.06\ty=1997.38 \nLabel=Strip\t611\tX=103221.79\ty=2073.35 \nLabel=Strip\t612\tX=103571.34\ty=2164.90 \nLabel=Strip\t613\tX=103221.05\ty=2240.75 \nLabel=Strip\t614\tX=103570.57\ty=2332.42 \nLabel=Strip\t615\tX=103220.26\ty=2408.15 \nLabel=Strip\t616\tX=103569.74\ty=2499.94 \nLabel=Strip\t617\tX=103219.40\ty=2575.55 \nLabel=Strip\t618\tX=103568.85\ty=2667.46 \nLabel=Strip\t619\tX=103218.49\ty=2742.95 \nLabel=Strip\t620\tX=103567.91\ty=2834.98 \nLabel=Strip\t621\tX=103217.51\ty=2910.36 \nLabel=Strip\t622\tX=103566.91\ty=3002.51 \nLabel=Strip\t623\tX=103216.49\ty=3077.76 \nLabel=Strip\t624\tX=103565.85\ty=3170.03 \nLabel=Strip\t625\tX=103215.40\ty=3245.16 \nLabel=Strip\t626\tX=103564.73\ty=3337.55 \nLabel=Strip\t627\tX=103214.26\ty=3412.57 \nLabel=Strip\t628\tX=103563.55\ty=3505.08 \nLabel=Strip\t629\tX=103213.06\ty=3579.97 \nLabel=Strip\t630\tX=103562.32\ty=3672.61 \nLabel=Strip\t631\tX=103211.80\ty=3747.38 \nLabel=Strip\t632\tX=103561.03\ty=3840.13 \nLabel=Strip\t633\tX=103210.48\ty=3914.79 \nLabel=Strip\t634\tX=103559.68\ty=4007.66 \nLabel=Strip\t635\tX=103209.11\ty=4082.19 \nLabel=Strip\t636\tX=103558.28\ty=4175.19 \nLabel=Strip\t637\tX=103207.68\ty=4249.60 \nLabel=Strip\t638\tX=103556.81\ty=4342.71 \nLabel=Strip\t639\tX=103206.19\ty=4417.01 \nLabel=Strip\t640\tX=103555.29\ty=4510.24 \nLabel=Strip\t641\tX=103204.64\ty=4584.42 \nLabel=Strip\t642\tX=103553.72\ty=4677.77 \nLabel=Strip\t643\tX=103203.04\ty=4751.65 \nLabel=Strip\t644\tX=103552.08\ty=4845.30 \nLabel=Strip\t645\tX=103201.38\ty=4919.24 \nLabel=Strip\t646\tX=103550.39\ty=5012.83 \nLabel=Strip\t647\tX=103199.66\ty=5086.65 \nLabel=Strip\t648\tX=103548.64\ty=5180.36 \nLabel=Strip\t649\tX=103197.88\ty=5254.06 \nLabel=Strip\t650\tX=103546.83\ty=5347.89 \nLabel=Strip\t651\tX=103196.05\ty=5421.47 \nLabel=Strip\t652\tX=103544.96\ty=5515.42 \nLabel=Strip\t653\tX=103194.16\ty=5588.88 \nLabel=Strip\t654\tX=103543.04\ty=5682.95 \nLabel=Strip\t655\tX=103192.21\ty=5756.29 \nLabel=Strip\t656\tX=103541.06\ty=5850.49 \nLabel=Strip\t657\tX=103190.21\ty=5923.70 \nLabel=Strip\t658\tX=103539.02\ty=6018.02 \nLabel=Strip\t659\tX=103188.14\ty=6091.11 \nLabel=Strip\t660\tX=103536.92\ty=6185.55 \nLabel=Strip\t661\tX=103186.02\ty=6258.53 \nLabel=Strip\t662\tX=103534.77\ty=6353.08 \nLabel=Strip\t663\tX=103183.84\ty=6425.94 \nLabel=Strip\t664\tX=103532.56\ty=6520.62 \nLabel=Strip\t665\tX=103181.61\ty=6593.35 \nLabel=Strip\t666\tX=103530.29\ty=6688.15 \nLabel=Strip\t667\tX=103179.31\ty=6760.77 \nLabel=Strip\t668\tX=103527.96\ty=6855.69 \nLabel=Strip\t669\tX=103176.96\ty=6928.18 \nLabel=Strip\t670\tX=103525.58\ty=7023.22 \nLabel=Strip\t671\tX=103174.55\ty=7095.59 \nLabel=Strip\t672\tX=103523.14\ty=7190.75 \nLabel=Strip\t673\tX=103172.09\ty=7263.01 \nLabel=Strip\t674\tX=103520.64\ty=7358.29 \nLabel=Strip\t675\tX=103169.56\ty=7430.42 \nLabel=Strip\t676\tX=103518.08\ty=7525.82 \nLabel=Strip\t677\tX=103166.98\ty=7597.84 \nLabel=Strip\t678\tX=103515.47\ty=7693.36 \nLabel=Strip\t679\tX=103164.34\ty=7765.25 \nLabel=Strip\t680\tX=103512.80\ty=7860.89 \nLabel=Strip\t681\tX=103161.65\ty=7932.67 \nLabel=Strip\t682\tX=103510.07\ty=8028.43 \nLabel=Strip\t683\tX=103158.89\ty=8100.08 \nLabel=Strip\t684\tX=103507.28\ty=8195.96 \nLabel=Strip\t685\tX=103156.08\ty=8267.50 \nLabel=Strip\t686\tX=103504.44\ty=8363.50 \nLabel=Strip\t687\tX=103153.21\ty=8434.91 \nLabel=Strip\t688\tX=103501.54\ty=8531.03 \nLabel=Strip\t689\tX=103150.29\ty=8602.33 \nLabel=Strip\t690\tX=103498.58\ty=8698.57 \nLabel=Strip\t691\tX=103147.30\ty=8769.74 \nLabel=Strip\t692\tX=103495.56\ty=8866.10 \nLabel=Strip\t693\tX=103144.26\ty=8937.16 \nLabel=Strip\t694\tX=103492.49\ty=9033.64 \nLabel=Strip\t695\tX=103141.16\ty=9104.57 \nLabel=Strip\t696\tX=103489.35\ty=9201.17 \nLabel=Strip\t697\tX=103138.00\ty=9271.99 \nLabel=Strip\t698\tX=103486.16\ty=9368.71 \nLabel=Strip\t699\tX=103134.79\ty=9439.40 \nLabel=Strip\t700\tX=103482.92\ty=9536.24 \nLabel=Strip\t701\tX=103131.52\ty=9606.82 \nLabel=Strip\t702\tX=103479.61\ty=9703.78 \nLabel=Strip\t703\tX=103128.19\ty=9774.23 \nLabel=Strip\t704\tX=103476.25\ty=9871.31 \nLabel=Strip\t705\tX=103124.80\ty=9941.64 \nLabel=Strip\t706\tX=103472.83\ty=10038.85 \nLabel=Strip\t707\tX=103121.36\ty=10109.06 \nLabel=Strip\t708\tX=103469.35\ty=10206.38 \nLabel=Strip\t709\tX=103117.86\ty=10276.47 \nLabel=Strip\t710\tX=103465.81\ty=10373.91 \nLabel=Strip\t711\tX=103114.30\ty=10443.89 \nLabel=Strip\t712\tX=103462.22\ty=10541.45 \nLabel=Strip\t713\tX=103110.68\ty=10611.30 \nLabel=Strip\t714\tX=103458.57\ty=10708.98 \nLabel=Strip\t715\tX=103107.01\ty=10778.72 \nLabel=Strip\t716\tX=103454.86\ty=10876.52 \nLabel=Strip\t717\tX=103103.27\ty=10946.13 \nLabel=Strip\t718\tX=103451.10\ty=11044.05 \nLabel=Strip\t719\tX=103099.48\ty=11113.54 \nLabel=Strip\t720\tX=103447.27\ty=11211.58 \nLabel=Strip\t721\tX=103095.64\ty=11280.95 \nLabel=Strip\t722\tX=103443.39\ty=11379.12 \nLabel=Strip\t723\tX=103091.73\ty=11448.37 \nLabel=Strip\t724\tX=103439.45\ty=11546.65 \nLabel=Strip\t725\tX=103087.77\ty=11615.78 \nLabel=Strip\t726\tX=103435.46\ty=11714.18 \nLabel=Strip\t727\tX=103083.75\ty=11783.19 \nLabel=Strip\t728\tX=103431.41\ty=11881.71 \nLabel=Strip\t729\tX=103079.67\ty=11950.60 \nLabel=Strip\t730\tX=103427.29\ty=12049.24 \nLabel=Strip\t731\tX=103075.54\ty=12118.01 \nLabel=Strip\t732\tX=103423.13\ty=12216.77 \nLabel=Strip\t733\tX=103071.35\ty=12285.43 \nLabel=Strip\t734\tX=103418.90\ty=12384.30 \nLabel=Strip\t735\tX=103067.10\ty=12452.84 \nLabel=Strip\t736\tX=103414.62\ty=12551.84 \nLabel=Strip\t737\tX=103062.79\ty=12620.25 \nLabel=Strip\t738\tX=103410.27\ty=12719.37 \nLabel=Strip\t739\tX=103058.42\ty=12787.65 \nLabel=Strip\t740\tX=103405.87\ty=12886.89 \nLabel=Strip\t741\tX=103054.00\ty=12955.06 \nLabel=Strip\t742\tX=103401.42\ty=13054.42 \nLabel=Strip\t743\tX=103049.52\ty=13122.47 \nLabel=Strip\t744\tX=103396.90\ty=13221.95 \nLabel=Strip\t745\tX=103044.98\ty=13289.88 \nLabel=Strip\t746\tX=103392.33\ty=13389.48 \nLabel=Strip\t747\tX=103040.39\ty=13457.29 \nLabel=Strip\t748\tX=103387.70\ty=13557.01 \nLabel=Strip\t749\tX=103035.74\ty=13624.70 \nLabel=Strip\t750\tX=103383.01\ty=13724.53 \nLabel=Strip\t751\tX=103031.03\ty=13792.10 \nLabel=Strip\t752\tX=103378.27\ty=13892.06 \nLabel=Strip\t753\tX=103026.26\ty=13959.51 \nLabel=Strip\t754\tX=103373.47\ty=14059.58 \nLabel=Strip\t755\tX=103021.43\ty=14126.91 \nLabel=Strip\t756\tX=103368.61\ty=14227.11 \nLabel=Strip\t757\tX=103016.55\ty=14294.32 \nLabel=Strip\t758\tX=103363.69\ty=14394.63 \nLabel=Strip\t759\tX=103011.61\ty=14461.72 \nLabel=Strip\t760\tX=103358.72\ty=14562.16 \nLabel=Strip\t761\tX=103006.61\ty=14629.12 \nLabel=Strip\t762\tX=103353.68\ty=14729.68 \nLabel=Strip\t763\tX=103001.55\ty=14796.53 \nLabel=Strip\t764\tX=103348.59\ty=14897.20 \nLabel=Strip\t765\tX=102996.44\ty=14963.93 \nLabel=Strip\t766\tX=103343.45\ty=15064.72 \nLabel=Strip\t767\tX=102991.27\ty=15131.33 \nLabel=Strip\t768\tX=103338.24\ty=15232.25 \nLabel=Strip\t769\tX=102986.04\ty=15298.73 \nLabel=Strip\t770\tX=103332.98\ty=15399.76 \nLabel=Strip\t771\tX=102980.76\ty=15466.13 \nLabel=Strip\t772\tX=103327.66\ty=15567.28 \nLabel=Strip\t773\tX=102975.41\ty=15633.53 \nLabel=Strip\t774\tX=103322.28\ty=15734.80 \nLabel=Strip\t775\t
